vi "Create (Factory).vi"(5 "Sequencing":refnum<class "MessageQ.lvclass">, 6 "Variables":refnum<class "Variables.lvclass">, 7 "VolatusAPI":refnum<class "VolatusAPI.lvclass">, 8 "error in (no error)":refnum<class "MultiErrors.lvclass">, 10 "Condition Config":refnum<class "Condition Config.lvclass">) -> (0 "error out":refnum<class "MultiErrors.lvclass">, 3 "Condition out":refnum<class "Condition.lvclass">)   [LabVIEW 2020, in "VolatusSeq.lvlib" / "Condition.lvclass"]
uses:
  Condition.lvclass
  VolatusErrorUtilities/MultiErrors/MultiErrors.lvclass
  Volatus/VolatusAPI/VolatusAPI.lvclass
  VolatusSeqConfig/Condition Config/Condition Config.lvclass
  Volatus/MessageQ/MessageQ.lvclass
  Variables/Variables.lvclass
  VolatusErrorUtilities/MultiErrors/MultiErrors.lvclass/MultiErrors.ctl
  VolatusErrorUtilities/MultiErrors/Last Error to Wire.vi
  Condition.lvclass/Condition.ctl
  VolatusSeq.lvlib
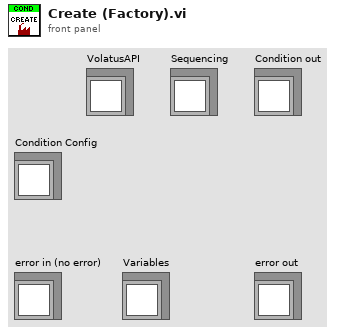
[diagram p1: front panel]
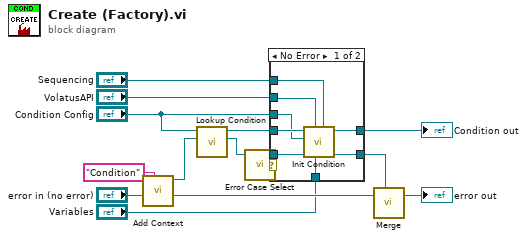
[diagram p0: block diagram]
diagram:
  n1 = call "Add Context.vi"("Context"="Condition", "MultiErrors in"="error in (no error)") -> ("Original Context"=w7:refnum<class "MultiErrors.lvclass">, "Added Context"=w5:refnum<class "MultiErrors.lvclass">)  [unwired: 8 in]
  n2 = call "Lookup Condition.vi"("error in (no error)"=w5, "Condition Config"="Condition Config") -> ("error out"=w9:refnum<class "MultiErrors.lvclass">, "Condition"=w15:refnum<class "Condition.lvclass">)  [unwired: 8 in]
  n3 = call "Error Case Select.vi"("MultiErrors in"=w9) -> ("MultiErrors out"=w10:refnum<class "MultiErrors.lvclass">, "error out"=w11:errorcluster)  [unwired: 7 in]
  n4 = case shown="No Error" w11 {
    tunnel: w15 -> [w23 _]
    tunnel: "Condition Config" -> [w21 _]
    tunnel: "VolatusAPI" -> [w22 _]
    tunnel: [w20 _] -> w12
    tunnel: w10 -> [w19 w24]
    tunnel: [w18 w24] -> w3
    tunnel: "Sequencing" -> [w17 _]
    tunnel: "Variables" -> [w16 _]
    frame No Error {
      n5 = call-dynamic "Init Condition.vi"("Sequencing"=w17, "Variables"=w16, "VolatusAPI"=w22, "error in (no error)"=w19, "Condition Config"=w21, "Condition in"=w23) -> ("error out"=w18:refnum<class "MultiErrors.lvclass">, "Condition out"=w20:refnum<class "Condition.lvclass">)  [unwired: 4 in]
    }
    frame Error {
    }
  }
  "Condition out" <- w12
  n6 = call "Merge.vi"("First Error In"=w7, "Second Error In"=w3) -> ("MultiErrors out"=→"error out":refnum<class "MultiErrors.lvclass">)  [unwired: 5 in]
